vi "Factory Core.vi"(8 "error in (no error)":errorcluster, 11 "Factory Plugin Framework in":refnum<class "Factory Plugin Framework.lvclass">=refnum) -> (0 "error out":errorcluster, 3 "Factory Plugin Framework out":refnum<class "Factory Plugin Framework.lvclass">)   [LabVIEW 2018, in "Factory Plugin Framework.lvlib" / "Factory Plugin Framework.lvclass"]
uses:
  Factory Plugin Framework.lvclass
  Factory Plugin Framework.lvclass/Factory Plugin Framework.ctl
  Accessors/Read Loaded Plugins.vi
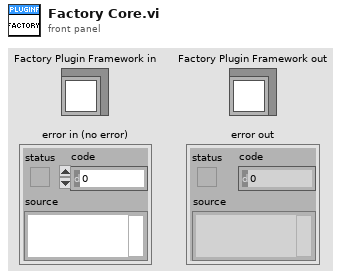
[diagram p1: front panel]
types:
  T1 = cluster{"Plugin Name":string, "Plugin Object":refnum<class>}[]
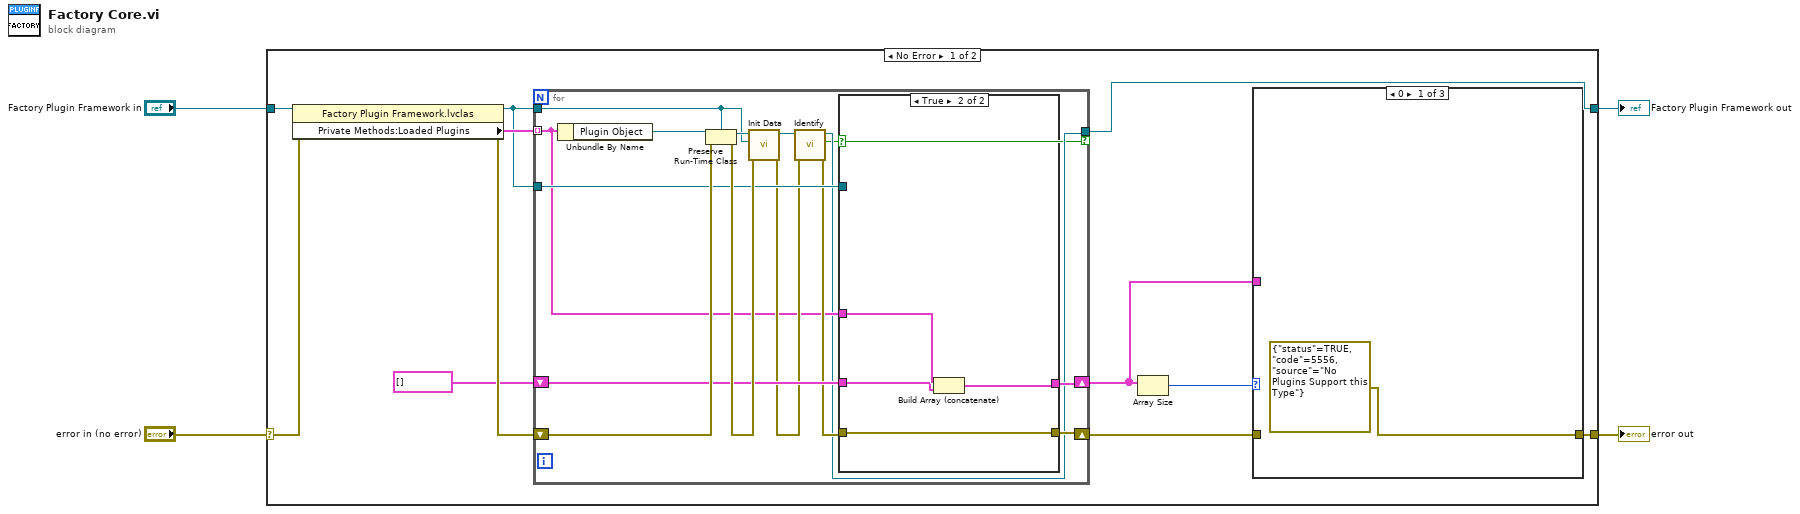
[diagram p0: block diagram]
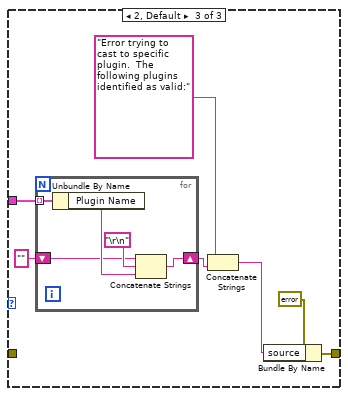
[diagram p3: hidden frame]
diagram:
  n1 = case shown="No Error" "error in (no error)" {
    selector: "error in (no error)" -> [w15 w52]
    tunnel: [w11 w52] -> w3
    tunnel: [w5 w51] -> w1
    tunnel: "Factory Plugin Framework in" -> [w6 w51]
    frame No Error {
      n2 = property class="Factory Plugin Framework.lvclas"(reference=w6, error in=w15) -> (reference out=w7:refnum<class "Factory Plugin Framework.lvclass">, error out=w13:errorcluster, "Private Methods:Loaded Plugins"=w14:T1)
      n3 = for {
        tunnel: w7 -> [w34]
        tunnel: w14 -> [w32] mode=indexing
        shift-right: [w39] -> w12
        shift-left: w13 -> [w44]
        tunnel: w7 -> [w41]
        shift-right: [w38] -> w8
        shift-left: T1 [] -> [w42]
        tunnel: [w31] -> w5 if=w30
        n4 = Unbundle By Name(w32) -> ("Plugin Object"=w33:refnum<class>)
        n5 = Preserve Run-Time Class(object in=w33, error in=w44, 2:w34) -> (object out=w36:refnum<class "Factory Plugin Framework.lvclass">, error out=w43:errorcluster)
        n6 = call-dynamic "Init Data.vi"("error in (no error)"=w43, "Data Object"=w34, "Factory Plugin Framework in"=w36) -> ("error out"=w37:errorcluster, "Factory Plugin Framework out"=w35:refnum<class "Factory Plugin Framework.lvclass">)  [unwired: 7 in]
        n7 = call-dynamic "Identify.vi"("error in (no error)"=w37, "Factory Plugin Framework in"=w35) -> ("error out"=w40:errorcluster, "Plugin is Valid"=w30:bool, "Factory Plugin Framework out"=w31:refnum<class "Factory Plugin Framework.lvclass">)  [unwired: 7 in]
        n8 = case shown="True" w30 {
          tunnel: w42 -> [w45 w48]
          tunnel: w41 -> [_ _]
          tunnel: w40 -> [w46 w50]
          tunnel: [w46 w50] -> w39
          tunnel: [w45 w47] -> w38
          tunnel: w32 -> [_ w49]
          frame False {
          }
          frame True {
            n9 = Build Array (concatenate)(w49, w48) -> (w47:T1)
          }
        }
      }
      n10 = Array Size(array=w8) -> (size(s)=w9:i32)
      n11 = case shown="0" w9 {
        tunnel: w12 -> [_ w17 _]
        tunnel: [errorcluster {"status"=TRUE, "code"=5556, "source"="No Plugins Support this Type"} ("error out") w17 w22] -> w11
        tunnel: w8 -> [_ _ w24]
        frame 0 {
        }
        frame 1 {
        }
        frame 2, Default {
          n12 = for {
            tunnel: w24 -> [w29] mode=indexing
            shift-right: [w26] -> w19
            shift-left: "" -> [w25]
            n13 = Unbundle By Name(w29) -> ("Plugin Name"=w28:string)
            n14 = Concatenate Strings(w25, "\r\n", w28) -> (w26:string)
          }
          n15 = Concatenate Strings("Error trying to cast to specific plugin.  The following plugins identified as valid:", w19) -> (w18:string)
          n16 = Bundle By Name(cluster=errorcluster {"status"=TRUE, "code"=5557, "source"=""} ("error out"), "source"=w18) -> (w22:errorcluster)
        }
      }
    }
    frame Error {
    }
  }
  "error out" <- w3
  "Factory Plugin Framework out" <- w1
